vi "新剖面数据组合.vi"(10 "columns":string[](array[string]), 11 "剖面数据":string[][](array[string])) -> (3 "结果字符串":string)   [LabVIEW 2016, in "数据传输系统-02.lvlib"]
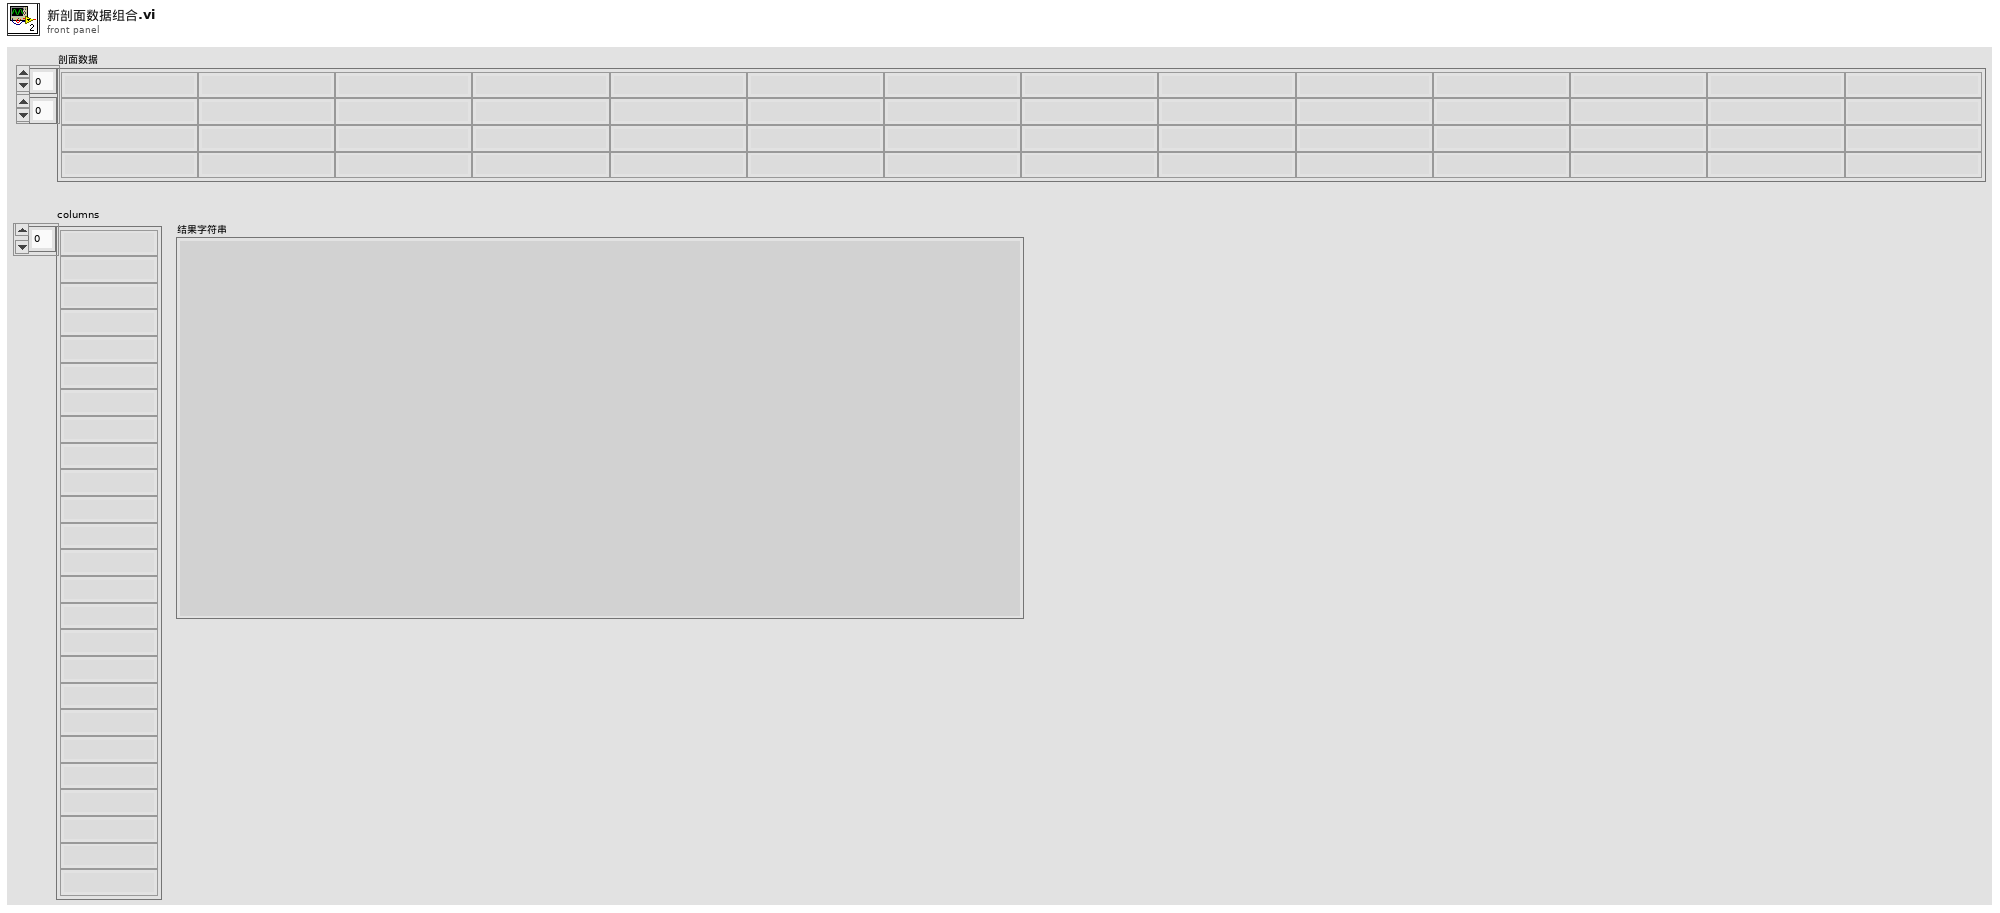
[diagram p1: front panel]
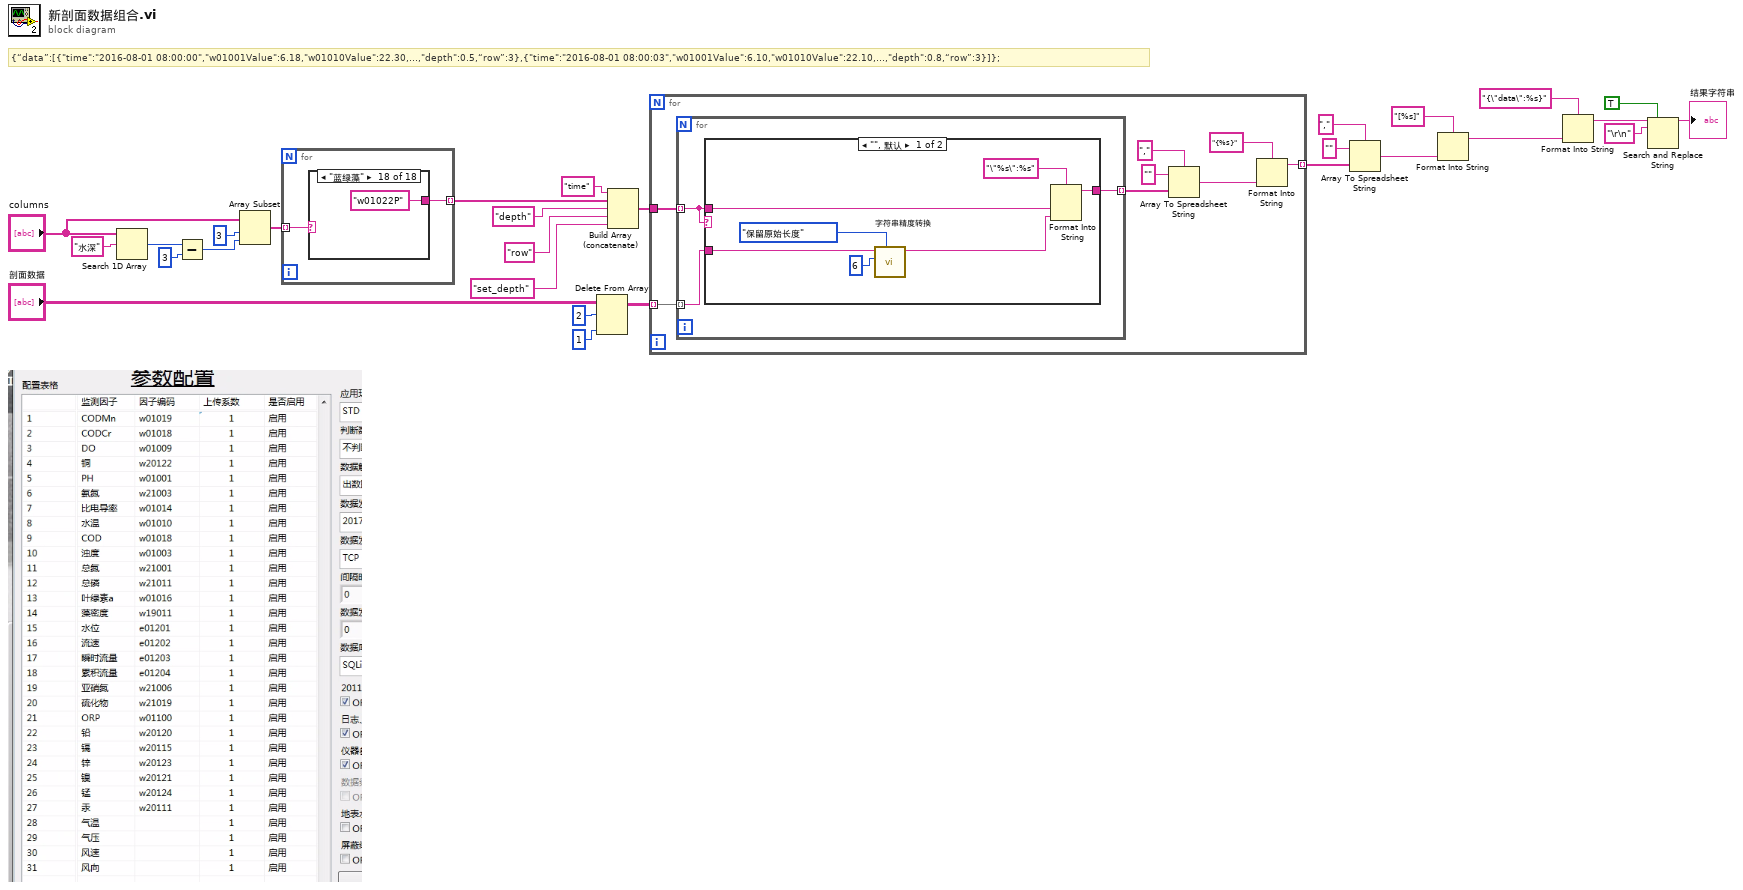
[diagram p0: block diagram]
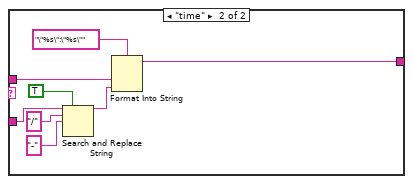
[diagram p2: hidden frame]
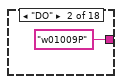
[diagram p4: hidden frame]
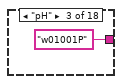
[diagram p5: hidden frame]
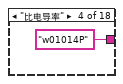
[diagram p6: hidden frame]
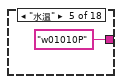
[diagram p7: hidden frame]
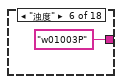
[diagram p8: hidden frame]
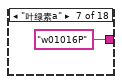
[diagram p9: hidden frame]
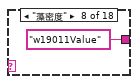
[diagram p10: hidden frame]
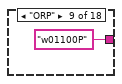
[diagram p11: hidden frame]
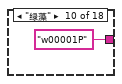
[diagram p12: hidden frame]
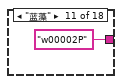
[diagram p13: hidden frame]
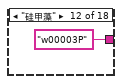
[diagram p14: hidden frame]
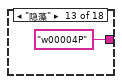
[diagram p15: hidden frame]
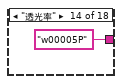
[diagram p16: hidden frame]
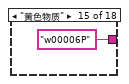
[diagram p17: hidden frame]
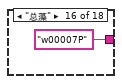
[diagram p18: hidden frame]
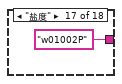
[diagram p19: hidden frame]
diagram:
  # "{“data”:[{\"time\":\"2016-08-01 08:00:00\",\"w01001Value\":6.18,\"w01010Value\":22.30,…,\"depth\":0.5,“row”:3},{\"time\":\"2016-08-01 08:00:03\",\"w01001Value\":6.10,\"w01010Value\":22.10,…,\"depth\":0.8,“row”:3}]};"
  n1 = Search 1D Array(1D array="columns", element="水深" ("元素")) -> (index of element=w18:i32)  [unwired: 1 in]
  n2 = Subtract(x=w18, y=3) -> (x-y=w24:i32)
  n3 = Array Subset(array="columns", index=3 ("索引"), length=w24) -> (w25:string[])
  n4 = for {
    tunnel: w25 -> [w30] mode=indexing
    tunnel: [w29] -> w22 mode=indexing
    n5 = case shown="\"蓝绿藻\"" w30 {
      tunnel: [_ "w01009P" "w01001P" "w01014P" "w01010P" "w01003P" "w01016P" "w19011Value" "w01100P" "w00001P" "w00002P" "w00003P" "w00004P" "w00005P" "w00006P" "w00007P" "w01002P" "w01022P"] -> w29
      frame "", Default {
      }
      frame "DO" {
      }
      frame "pH" {
      }
      frame "比电导率" {
      }
      frame "水温" {
      }
      frame "浊度" {
      }
      frame "叶绿素a" {
      }
      frame "藻密度" {
      }
      frame "ORP" {
      }
      frame "绿藻" {
      }
      frame "蓝藻" {
      }
      frame "硅甲藻" {
      }
      frame "隐藻" {
      }
      frame "透光率" {
      }
      frame "黄色物质" {
      }
      frame "总藻" {
      }
      frame "盐度" {
      }
      frame "蓝绿藻" {
      }
    }
  }
  n6 = Delete From Array(array="剖面数据", length=2 ("长度"), index (col)=1 ("禁用的索引 (列)")) -> (array with subset deleted=w4:string[][])  [unwired: 1 in, 1 out]
  n7 = Build Array (concatenate)("time" ("元素"), w22, "depth" ("元素"), "row" ("元素"), "set_depth" ("元素")) -> (w21:string[])
  n8 = for {
    tunnel: w4 -> [w54] mode=indexing
    tunnel: w21 -> [w55]
    tunnel: [w49] -> w15 mode=indexing
    n9 = for {
      tunnel: w55 -> [w57] mode=indexing
      tunnel: w54 -> [w56] mode=indexing
      tunnel: [w58] -> w51 mode=indexing
      n10 = case shown="\"\", 默认" w57 {
        tunnel: [w64 w72] -> w58
        tunnel: w57 -> [w63 w71]
        tunnel: w56 -> [w62 w67]
        frame "", Default {
          n11 = call "字符串精度转换.vi"("枚举"=enum16{"小数位修约", "保留原始长度"}."保留原始长度", "数据精度"=6, "输入字符串"=w62) -> ("输出字符串"=w59:string)  [unwired: 7 in, 1 out]
          n12 = Format Into String(format string="\"%s\":%s" ("格式字符串"), w63, w59) -> (resulting string=w64:string)  [unwired: 2 in, 1 out]
        }
        frame "time" {
          n13 = Search and Replace String(replace all?=TRUE ("替换全部？(F)"), input string=w67, search string="/" ("搜索字符串"), replace string="-" ("替换字符串(\"\")")) -> (result string=w66:string)  [unwired: 4 in, 3 out]
          n14 = Format Into String(format string="\"%s\":\"%s\"" ("格式字符串"), w71, w66) -> (resulting string=w72:string)  [unwired: 2 in, 1 out]
        }
      }
    }
    n15 = Array To Spreadsheet String(delimiter (Tab)="," ("分隔符(Tab)"), array=w51, 3:"" ("格式字符串")) -> (spreadsheet string=w48:string)
    n16 = Format Into String(format string="{%s}" ("格式字符串"), w48) -> (resulting string=w49:string)  [unwired: 2 in, 1 out]
  }
  n17 = Array To Spreadsheet String(delimiter (Tab)="," ("分隔符(Tab)"), array=w15, 3:"" ("格式字符串")) -> (spreadsheet string=w11:string)
  n18 = Format Into String(format string="[%s]" ("格式字符串"), w11) -> (resulting string=w12:string)  [unwired: 2 in, 1 out]
  n19 = Format Into String(format string="{\"data\":%s}" ("格式字符串"), w12) -> (resulting string=w8:string)  [unwired: 2 in, 1 out]
  n20 = Search and Replace String(replace all?=TRUE ("替换全部？(F)"), input string=w8, search string="\r\n") -> (result string=→"结果字符串":string)  [unwired: 5 in, 3 out]
